vi "for loop.vi"() -> ()   [LabVIEW 2012]
panel:
  out "Array":dbl[](array[numeric])
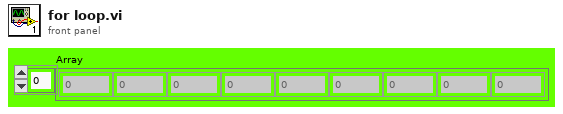
[diagram p1: front panel]
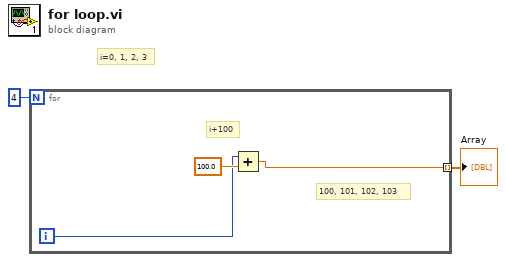
[diagram p0: block diagram]
diagram:
  # "i=0, 1, 2, 3"
  n1 = for {
    N: 4 -> [_]
    tunnel: [w3] -> w1 mode=indexing
    i -> [w4]
    # "100, 101, 102, 103"
    # "i+100"
    n2 = Add(x=w4, y=100.0) -> (x+y=w3:dbl)
  }
  "Array" <- w1
